vi "sub parse frame bp.vi"(8 "error in (no error)":errorcluster, 11 "<bp> String":string="   <bp x 56.88426948876875 y 39.15890324252262 bp>") -> (0 "error out":errorcluster, 3 "bp data":T1)   [LabVIEW 2018, in "Frame Analizer.lvclass"]
uses:
  Frame Analizer.lvclass
  frame bp data.ctl
panel:
  out "output 4":string
  out "output 1":string
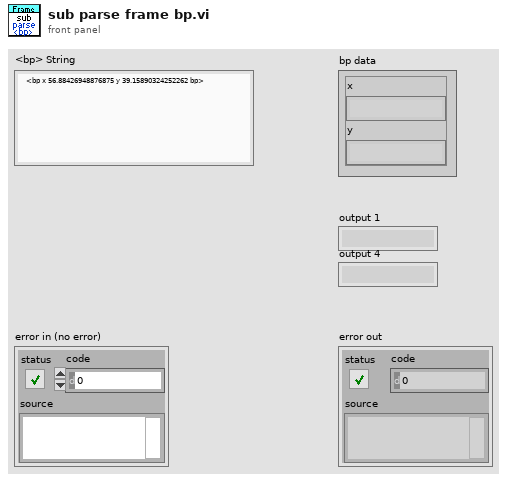
[diagram p1: front panel]
types:
  T1 = typedef "Frame Analizer.lvclass/frame bp data.ctl" = cluster{"x":string, "y":string}
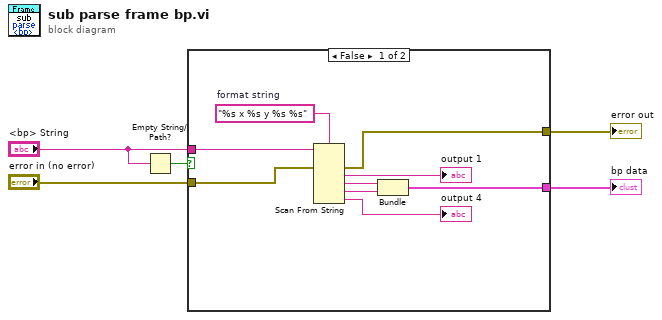
[diagram p0: block diagram]
diagram:
  n1 = Empty String/Path?(string/path="<bp> String") -> (empty?=w1:bool)
  n2 = case shown="False" w1 {
    tunnel: [w9 _] -> w5
    tunnel: "error in (no error)" -> [w8 w15]
    tunnel: [w7 w15] -> w3
    tunnel: "<bp> String" -> [w6 _]
    frame False {
      w14 = "%s x %s y %s %s"  # format string
      n3 = Scan From String(format string=w14, input string=w6, error in=w8) -> (error out=w7:errorcluster, output 1=→"output 1":string, output 2=w11:string, output 3=w10:string, output 4=→"output 4":string)  [unwired: 5 in, 2 out]
      n4 = Bundle(w11, w10) -> (w9:cluster{string, string})  [unwired: 1 in]
    }
    frame True {
    }
  }
  "bp data" <- w5
  "error out" <- w3
